vi "MCCETC_Global.vi"() -> ()   [LabVIEW 2019]
panel:
  out "MCCETC03_T7":dbl
  out "MCCETC03_T6":dbl
  out "MCCETC03_T5":dbl
  out "MCCETC03_T4":dbl
  out "MCCETC03_T3":dbl
  out "MCCETC03_T2":dbl
  out "MCCETC03_T1":dbl
  out "MCCETC03_ST":u32(colorbox)
  out "MCCETC03_T0":dbl
  out "MCCETC02_T7":dbl
  out "MCCETC02_T6":dbl
  out "MCCETC02_T5":dbl
  out "MCCETC02_T4":dbl
  out "MCCETC02_T3":dbl
  out "MCCETC02_T2":dbl
  out "MCCETC02_T1":dbl
  out "MCCETC02_ST":u32(colorbox)
  out "MCCETC02_T0":dbl
  out "MCCETC01_T7":dbl
  out "MCCETC01_T6":dbl
  out "MCCETC01_T5":dbl
  out "MCCETC01_T4":dbl
  out "MCCETC01_T3":dbl
  out "MCCETC01_T2":dbl
  out "MCCETC01_T1":dbl
  out "MCCETC01_ST":u32(colorbox)
  out "MCCETC01_T0":dbl
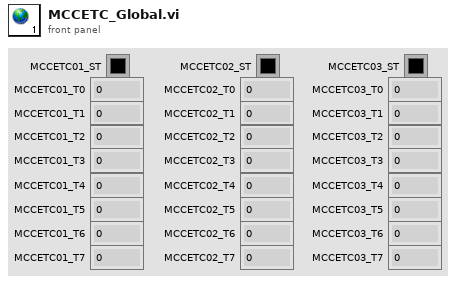
[diagram p1: front panel]
diagram:
